vi "Voltage Meas T12.vi"() -> ()   [LabVIEW 2021, in "Test Case T12.lvlib"]
uses:
  Test Case T12.lvlib
  NIDCpower/controls/Config.ctl
  NIDMM/LoadDMM t12.ctl
  NIDMM/Meas T12.ctl
  NIDCpower/NIDCPower T12.lvlib
panel:
  in  "Name 2":T1
  out "Name":T1
  in  "Load SMU":T2={"Range (Amps)"=0.2, "Resolution in Digits"=5.5} {"Resolution in Digits" items=["3 1/2"=3.5, "4 1/2"=4.5, "5 1/2"=5.5, "6 1/2"=6.5, "7 1/2"=7.5]; "Range (Amps)" format="%.2p"}
  in  "Cluster":T3={"Current Level"=0.01, "Current Level Range"=0.01, "Voltage Limit"=2.0, "Voltage Limit Range"=6.0, "Source Delay (Sec)"=0.1} {"Source Delay (Sec)" format="%.3p"; "Voltage Limit Range" format="%.5p"; "Voltage Limit" format="%.5p"; "Current Level Range" format="%.3p"; "Current Level" format="%.3p"}
  in  "Load DMM":refnum<k15>="Dev1"
  in  "error in":errorcluster
  out "error out":errorcluster
  in  "Load SMU Channel":string="0"
  in  "Load SMU":refnum<k15>="Dev1"
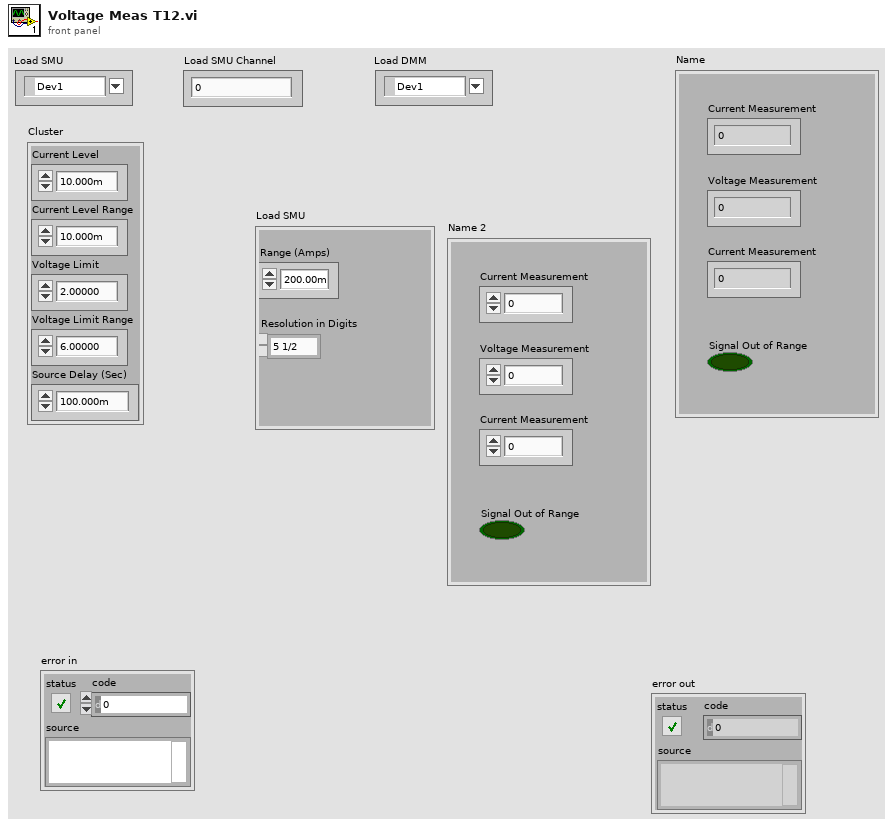
[diagram p1: front panel]
types:
  T1 = typedef "Meas T12.ctl" = cluster{"Current Measurement":dbl, "Voltage Measurement":dbl, "Signal Out of Range":bool, "Current in DMM":dbl}
  T2 = typedef "LoadDMM t12.ctl" = cluster{"Range (Amps)":dbl, "Resolution in Digits":dbl}
  T3 = typedef "NIDCPower T12.lvlib/Config.ctl" = cluster{"Current Level":dbl, "Current Level Range":dbl, "Voltage Limit":dbl, "Voltage Limit Range":dbl, "Source Delay (Sec)":dbl}
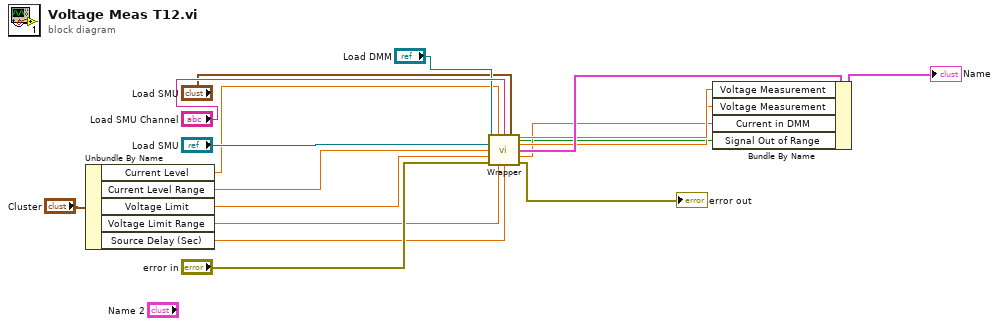
[diagram p0: block diagram]
diagram:
  n1 = Unbundle By Name("Cluster") -> ("Current Level"=w12:dbl, "Current Level Range"=w10:dbl, "Voltage Limit"=w11:dbl, "Voltage Limit Range"=w9:dbl, "Source Delay (Sec)"=w8:dbl)
  n2 = call "Wrapper.vi"("IVI Refnum in"="Load DMM", "Current Level"=w12, "Load SMU Channel"="Load SMU Channel", "Load SMU"="Load SMU", "Load SMU 2"="Load SMU", "Current Level Range"=w10, "Voltage Limit"=w11, "error in (no error)"="error in", "Voltage Limit Range"=w9, "Source Delay (Sec)"=w8) -> ("Numeric 2"=w4:dbl, "Numeric"=w3:dbl, "Name"=w6:T1, "Measurement"=w2:dbl, "Over Range?"=w1:bool, "error out"=→"error out":errorcluster)
  n3 = Bundle By Name(cluster=w6, "Voltage Measurement"=w4, "Voltage Measurement"=w3, "Current in DMM"=w2, "Signal Out of Range"=w1) -> (→"Name":T1)
